vi "AalborgDFCCommandDescriptors.vi"(4 "AalborgDFCCommand":T2="SetPoint") -> (0 "Error":bool, 1 "CommandDescriptorOutput":T1={"Command"="SetPoint", "Mnemonic"="S,", "Min"=0.0, "Max"=100.0, "ActionPath"=["CheckLimits", "PassCommand", "AssembleCommand", "Communicate", "ParseNumber", "Done"]})   [LabVIEW 2016]
uses:
  AalborgDFCCommand.ctl
  AalborgDFCCommandDescriptor.ctl
  AalborgDFCCommandPhases.ctl
panel:
  in  "CommandDescriptorArray":T1[](array[typedef])=[{"Command"="SetModeDigital", "Mnemonic"="M,D", "Min"=nan, "Max"=nan, "ActionPath"=["PassCommand", "Communicate", "CheckEcho", "Done"]}, {"Command"="SetModeAnalog", "Mnemonic"="M,A", "Min"=nan, "Max"=nan, "ActionPath"=["PassCommand", "Communicate", "CheckEcho", "Done"]}, {"Command"="ReadModeStatus", "Mnemonic"="M,S", "Min"=nan, "Max"=nan, "ActionPath"=["PassCommand", "Communicate", "ParseString", "Done"]}, {"Command"="SetPoint", "Mnemonic"="S", "Min"=0.0, "Max"=100.0, "ActionPath"=["CheckLimits", "PassCommand", "AssembleCommand", "Communicate", "CheckEcho", "ParseNumber", "Done"]}, {"Command"="FlowReading", "Mnemonic"="F", "Min"=nan, "Max"=nan, "ActionPath"=["PassCommand", "Communicate", "ParseNumber", "Done"]}, {"Command"="SetHighAlarm", "Mnemonic"="A,H", "Min"=0.0, "Max"=100.0, "ActionPath"=["CheckLimits", "PassCommand", "AssembleCommand", "Communicate", "Done"]}, {"Command"="SetLowAlarm", "Mnemonic"="A,L", "Min"=0.0, "Max"=100.0, "ActionPath"=["CheckLimits", "PassCommand", "AssembleCommand", "Communicate", "Done"]}, {"Command"="DisableAlarms", "Mnemonic"="A,D", "Min"=nan, "Max"=nan, "ActionPath"=["PassCommand", "Communicate", "Done"]}, {"Command"="ReadAlarmStatus", "Mnemonic"="A,S", "Min"=nan, "Max"=nan, "ActionPath"=["PassCommand", "Communicate", "Done"]}, {"Command"="FullScaleRatingSLPM", "Mnemonic"="E", "Min"=nan, "Max"=nan, "ActionPath"=["PassCommand", "Communicate", "ParseNumber", "Done"]}, {"Command"="ForceValveClosed", "Mnemonic"="V,C", "Min"=nan, "Max"=nan, "ActionPath"=["PassCommand", "Communicate", "CheckEcho", "Done"]}, {"Command"="ForceValveOpen", "Mnemonic"="V,O", "Min"=nan, "Max"=nan, "ActionPath"=["PassCommand", "Communicate", "CheckEcho", "Done"]}, {"Command"="SetValveAutomatic", "Mnemonic"="V,A", "Min"=nan, "Max"=nan, "ActionPath"=["PassCommand", "Communicate", "CheckEcho", "Done"]}, {"Command"="ValveStatus", "Mnemonic"="V,S", "Min"=nan, "Max"=nan, "ActionPath"=["PassCommand", "Communicate", "ParseString", "Done"]}, {"Command"="ReadAddress", "Mnemonic"="MR,7", "Min"=nan, "Max"=nan, "ActionPath"=["PassCommand", "Communicate", "ParseString", "Done"]}, {"Command"="ReadSerialNo", "Mnemonic"="MR,1", "Min"=nan, "Max"=nan, "ActionPath"=["PassCommand", "Communicate", "ParseString", "Done"]}, {"Command"="ReadModelNo", "Mnemonic"="MR,2", "Min"=nan, "Max"=nan, "ActionPath"=["PassCommand", "Communicate", "ParseString", "Done"]}, {"Command"="ReadFWVer", "Mnemonic"="MR,3", "Min"=nan, "Max"=nan, "ActionPath"=["PassCommand", "Communicate", "ParseString", "Done"]}, {"Command"="ReadFS", "Mnemonic"="MR,101", "Min"=nan, "Max"=nan, "ActionPath"=["PassCommand", "Communicate", "ParseNumber", "Done"]}, {"Command"="WriteAddress", "Mnemonic"="MW,7", "Min"=1.0, "Max"=255.0, "ActionPath"=["CheckLimits", "PassCommand", "AssembleCommand", "Communicate", "Done"]}]
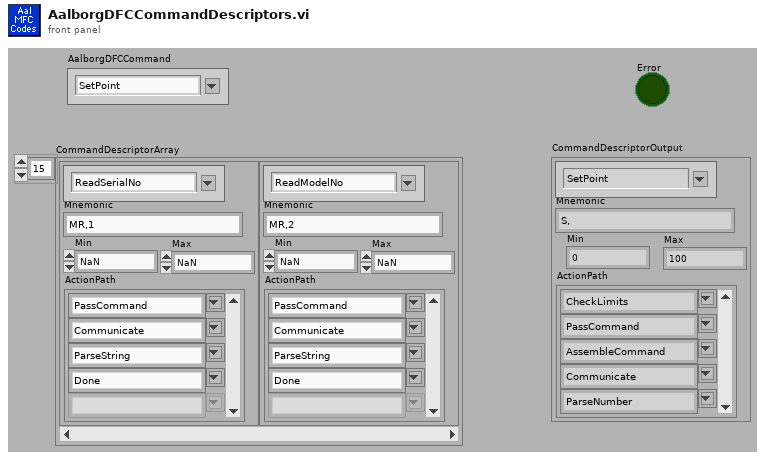
[diagram p1: front panel]
types:
  T1 = typedef "AalborgDFCCommandDescriptor.ctl" = cluster{"Command":T2, "Mnemonic":string, "Min":dbl, "Max":dbl, "ActionPath":T3[]}
  T2 = typedef "AalborgDFCCommand.ctl" = string
  T3 = typedef "AalborgDFCCommandPhases.ctl" = string
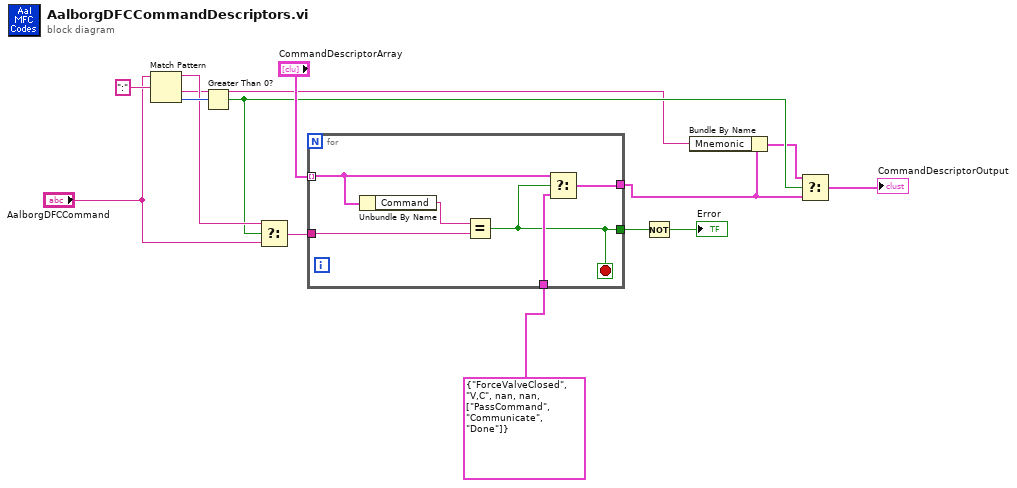
[diagram p0: block diagram]
diagram:
  n1 = Match Pattern(string="AalborgDFCCommand", regular expression=":") -> (before substring=w7:T2, after substring=w2:T2, offset past match=w10:i32)  [unwired: 2 out]
  n2 = Greater Than 0?(x=w10) -> (x > 0?=w5:bool)
  n3 = Select(t=w7, s=w5, f="AalborgDFCCommand") -> (s? t:f=w9:T2)
  n4 = for {
    tunnel: "CommandDescriptorArray" -> [w17] mode=indexing
    tunnel: w9 -> [w19]
    tunnel: [w18] -> w4
    tunnel: T1 {"Command"="ForceValveClosed", "Mnemonic"="V,C", "Min"=nan, "Max"=nan, "ActionPath"=["PassCommand", "Communicate", "Done"]} ("CommandDescriptor") -> [w16]
    tunnel: [w15] -> w13
    stop <- w15 stop-if-true
    n5 = Unbundle By Name(w17) -> ("Command"=w20:T2)
    n6 = Equal?(x=w20, y=w19) -> (x = y?=w15:bool)
    n7 = Select(t=w17, s=w15, f=w16) -> (s? t:f=w18:T1)
  }
  n8 = Not(x=w13) -> (.not. x?=→"Error":bool)
  n9 = Bundle By Name(cluster=w4, "Mnemonic"=w2) -> (w3:T1)
  n10 = Select(t=w3, s=w5, f=w4) -> (s? t:f=→"CommandDescriptorOutput":T1)
